vi "get_Components.vi"(0 "HGF_Composite":refnum<class "HGF_Composite.lvclass">, 5 "error in (no error)":errorcluster) -> (14 "dup HGF_Composite":refnum<class "HGF_Composite.lvclass">, 16 "Components":refnum<class "HGF_Component.lvclass">[](array[class]), 19 "error out":errorcluster)   [LabVIEW 2014, in "HGF_BaseClasses.lvlib" / "HGF_Composite.lvclass"]
doc: "Get a copy of Component array from Composite object."
uses:
  HGF_Composite.lvclass
  HGF_Component/HGF_Component.lvclass
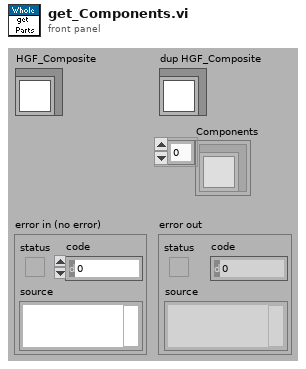
[diagram p1: front panel]
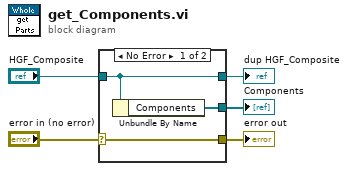
[diagram p0: block diagram]
diagram:
  n1 = case shown="No Error" "error in (no error)" {
    selector: "error in (no error)" -> [w8 w10]
    tunnel: [w8 w10] -> w4
    tunnel: [w7 w9] -> w2
    tunnel: "HGF_Composite" -> [w7 w9]
    tunnel: [w6 _] -> w1
    frame No Error {
      n2 = Unbundle By Name(w7) -> ("Components"=w6:refnum<class "HGF_Component.lvclass">[])
    }
    frame Error {
    }
  }
  "error out" <- w4
  "dup HGF_Composite" <- w2
  "Components" <- w1
